vi "Cleanup Proc.vi"   [LabVIEW 2020]
uses:
  bf27c383-259f-44cd-8351-e8a95deca1f4.vi
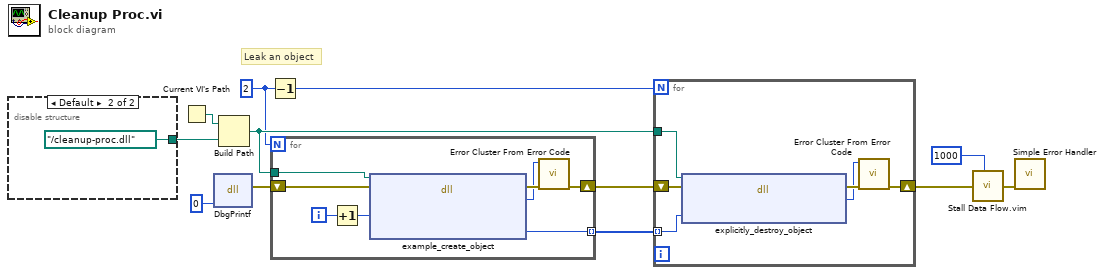
[diagram p0: block diagram]
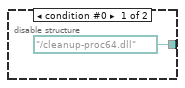
[diagram p2: hidden frame]
diagram:
  w2 = 2
  # "Leak an object"
  n1 = disable-structure shown="Default" {
    disable-tunnel: [path "../cleanup-proc64.dll" ("name or relative path") path "../cleanup-proc.dll" ("name or relative path")] -> w10
    frame condition #0 {
    }
    frame condition #1 (active) {
    }
  }
  n2 = Current VI's Path() -> (path=w11:path)
  n3 = dll-call lib="LabVIEW" fn="DbgPrintf"("NULL"=u64 0) -> (error out=w6:errorcluster)  [unwired: 5 in, 1 out]
  n4 = Build Path(base path=w11, name or relative path=w10) -> (appended path=w4:path)
  n5 = Decrement(x=w2) -> (x-1=w3:i32)
  n6 = for {
    N: w2 -> [_]
    shift-right: [w18] -> w9
    shift-left: w6 -> [w17]
    tunnel: [w16] -> w1 mode=indexing
    tunnel: w4 -> [w15]
    i -> [w20]
    n7 = Increment(x=w20) -> (x+1=w19:i32)
    n8 = dll-call lib="?" fn="example_create_object"(path in=w15, error in=w17, "Value"=w19) -> (error out=w22:errorcluster, "Err"=w21:i32, "Object-Pointer"=w16:u64)  [unwired: 3 in, 1 out]
    n9 = call <vilib>:"Error Cluster From Error Code.vi"("error in (no error)"=w22, "error code (0)"=w21) -> ("error out"=w18:errorcluster)  [unwired: 7 in]
  }
  n10 = for {
    N: w3 -> [_]
    shift-right: [w28] -> w12
    shift-left: w9 -> [w27]
    tunnel: w1 -> [w24] mode=indexing
    tunnel: w4 -> [w23]
    n11 = dll-call lib="?" fn="explicitly_destroy_object"(path in=w23, error in=w27, "Object-Pointer"=w24) -> (error out=w26:errorcluster, "Err"=w25:i32)  [unwired: 2 in, 1 out]
    n12 = call <vilib>:"Error Cluster From Error Code.vi"("error in (no error)"=w26, "error code (0)"=w25) -> ("error out"=w28:errorcluster)  [unwired: 7 in]
  }
  n13 = call "Stall Data Flow.vim"("value in"=w12, "milliseconds to wait"=u32 1000) -> ("value out"=w8:errorcluster)  [unwired: 1 out]
  n14 = call <vilib>:"Simple Error Handler.vi"("error in (no error)"=w8) -> ()  [unwired: 4 in, 5 out]
